vi "CRYConversion dB-Lin.vi"(4 "unit prefix":string, 5 "dB ref.":dbl=1.0 format="%#.12p", 6 "Log In array":dbl[](array[numeric]) format="%#.12p", 7 "Log In":dbl=94.0 format="%#.12p", 8 "Lin In array":dbl[](array[numeric]) format="%#.12p", 9 "Lin In":dbl=1.0 format="%#.12p") -> (0 "Lin Out array":dbl[](array[numeric]) format="%.2f", 1 "Lin Out":dbl=1002.374467254545 format="%.2f", 2 "Log Out array":dbl[](array[numeric]) format="%.2f", 3 "Log Out":dbl=33.979400086720375 format="%.2e")   [LabVIEW 2013]
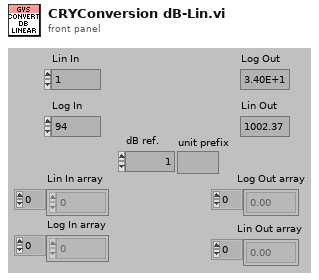
[diagram p1: front panel]
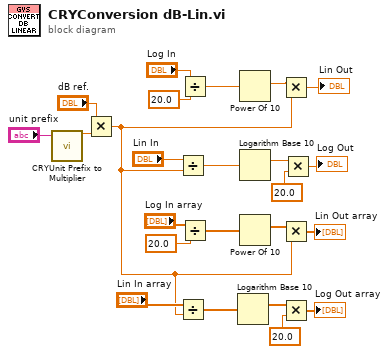
[diagram p0: block diagram]
diagram:
  n1 = call "CRYUnit Prefix to Multiplier.vi"("unit prefix"="unit prefix") -> ("multiplier"=w3:dbl)  [unwired: 4 out]
  n2 = Multiply(x="dB ref.", y=w3) -> (x*y=w2:dbl)
  n3 = Divide(x="Lin In", y=w2) -> (x/y=w1:dbl)
  n4 = Divide(x="Lin In array", y=w2) -> (x/y=w12:dbl[])
  n5 = Divide(x="Log In", y=20.0) -> (x/y=w24:dbl)
  n6 = Divide(x="Log In array", y=20.0) -> (x/y=w10:dbl[])
  n7 = Logarithm Base 10(1:w12) -> (0:w11:dbl[])
  n8 = Power Of 10(x=w24) -> (10^x=w18:dbl)
  n9 = Logarithm Base 10(1:w1) -> (0:w23:dbl)
  n10 = Power Of 10(x=w10) -> (10^x=w13:dbl[])
  n11 = Multiply(x=w18, y=w2) -> (x*y=→"Lin Out":dbl)
  n12 = Multiply(x=w13, y=w2) -> (x*y=→"Lin Out array":dbl[])
  n13 = Multiply(x=w11, y=20.0) -> (x*y=→"Log Out array":dbl[])
  n14 = Multiply(x=w23, y=20.0) -> (x*y=→"Log Out":dbl)
